vi "Receive Toveys.vi"(8 "error in (no error)":errorcluster, 11 "Model in":refnum<class "Model.lvclass">) -> (0 "error out":errorcluster, 2 "Data Received":bool, 3 "Model out":refnum<class "Model.lvclass">)   [LabVIEW 2016]
uses:
  Model.lvclass
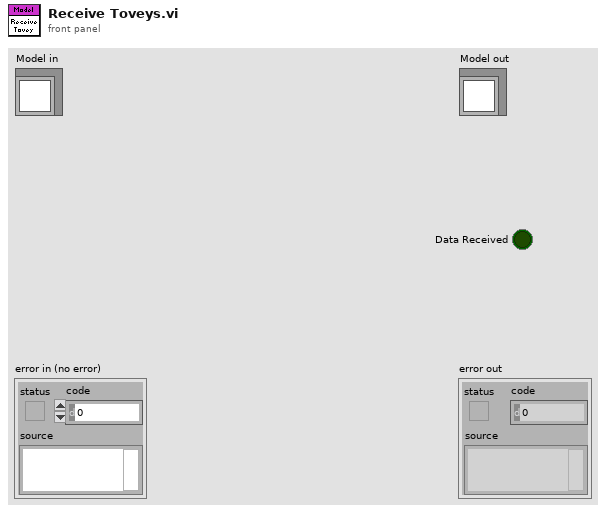
[diagram p1: front panel]
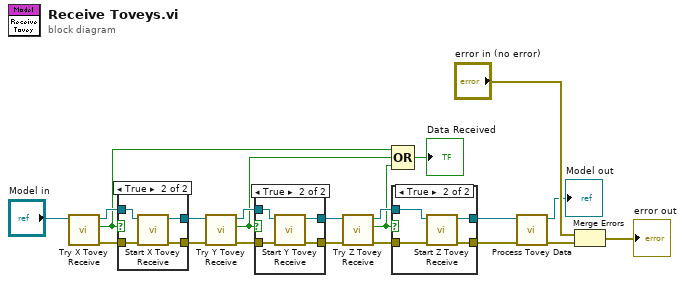
[diagram p0: block diagram]
diagram:
  n1 = call "Try X Tovey Receive.vi"("Model in"="Model in") -> ("error out"=w19:errorcluster, "Data Present"=w8:bool, "Model out"=w20:refnum<class "Model.lvclass">)  [unwired: 8 in]
  n2 = case shown="True" w8 {
    tunnel: w20 -> [w23 w27]
    tunnel: w19 -> [w22 w26]
    tunnel: [w23 w25] -> w16
    tunnel: [w22 w24] -> w15
    frame False {
    }
    frame True {
      n3 = call "Start X Tovey Receive.vi"("error in (no error)"=w26, "Model in"=w27) -> ("error out"=w24:errorcluster, "Model out"=w25:refnum<class "Model.lvclass">)  [unwired: 8 in]
    }
  }
  n4 = call "Try Y Tovey Receive.vi"("error in (no error)"=w15, "Model in"=w16) -> ("error out"=w17:errorcluster, "Data Present"=w7:bool, "Model out"=w18:refnum<class "Model.lvclass">)  [unwired: 7 in]
  n5 = case shown="True" w7 {
    tunnel: w18 -> [w29 w33]
    tunnel: w17 -> [w28 w32]
    tunnel: [w29 w31] -> w12
    tunnel: [w28 w30] -> w11
    frame False {
    }
    frame True {
      n6 = call "Start Y Tovey Receive.vi"("error in (no error)"=w32, "Model in"=w33) -> ("error out"=w30:errorcluster, "Model out"=w31:refnum<class "Model.lvclass">)  [unwired: 8 in]
    }
  }
  n7 = call "Try Z Tovey Receive.vi"("error in (no error)"=w11, "Model in"=w12) -> ("error out"=w13:errorcluster, "Data Present"=w6:bool, "Model out"=w14:refnum<class "Model.lvclass">)  [unwired: 7 in]
  n8 = Compound Arithmetic op=OR(w8, w7, w6) -> (→"Data Received":bool)
  n9 = case shown="True" w6 {
    tunnel: w14 -> [w34 w39]
    tunnel: w13 -> [w35 w38]
    tunnel: [w35 w37] -> w3
    tunnel: [w34 w36] -> w4
    frame False {
    }
    frame True {
      n10 = call "Start Z Tovey Receive.vi"("error in (no error)"=w38, "Model in"=w39) -> ("error out"=w37:errorcluster, "Model out"=w36:refnum<class "Model.lvclass">)  [unwired: 8 in]
    }
  }
  n11 = call "Process Tovey Data.vi"("error in (no error)"=w3, "Model in"=w4) -> ("error out"=w2:errorcluster, "Model out"=→"Model out":refnum<class "Model.lvclass">)  [unwired: 8 in]
  n12 = Merge Errors("error in (no error)", w2) -> (→"error out":errorcluster)
